vi "One Shot Button.vi"(11 "Button In":bool) -> (3 "Button Pressed?":bool)   [LabVIEW 2018]
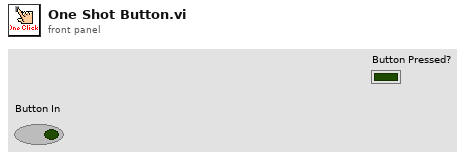
[diagram p1: front panel]
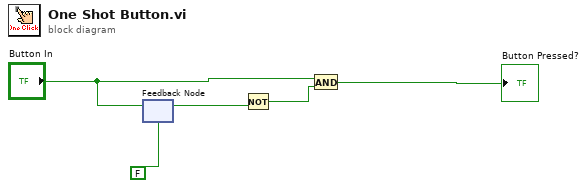
[diagram p0: block diagram]
diagram:
  n1 = feedback-in #1("Button In") -> ()
  n2 = feedback #1(FALSE) -> (w5:bool)
  n3 = Not(x=w5) -> (.not. x?=w2:bool)
  n4 = And(x="Button In", y=w2) -> (x .and. y?=→"Button Pressed?":bool)
